vi "DSF.Engine.Framework.Set Transceiver Count.vi"(10 "transceiver count":i32, 11 "Framework in":refnum<class "DSF.Engine.Framework.lvclass">) -> (3 "Framework out":refnum<class "DSF.Engine.Framework.lvclass">)   [LabVIEW 2017, in "Data Sharing Framework Engine.lvlib" / "DSF.Engine.Framework.lvclass"]
uses:
  DSF.Engine.Framework.lvclass
  DSF.Engine.Framework.lvclass/DSF.Engine.Framework.ctl
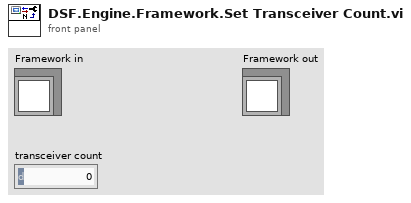
[diagram p1: front panel]
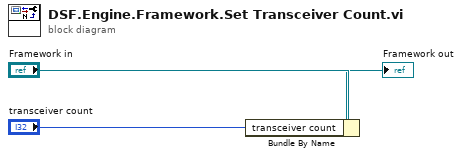
[diagram p0: block diagram]
diagram:
  n1 = Bundle By Name(cluster="Framework in", "transceiver count"="transceiver count") -> (→"Framework out":refnum<class "DSF.Engine.Framework.lvclass">)
